vi "WriteVSChSingleIncoming.vi"(7 "IncomingFRActive?":bool, 8 "error in (no error)":errorcluster, 10 "Output Refs":T1[](array[typedef]) format="%.0x", 11 "Refnum in":refnum<k21>) -> (0 "error out":errorcluster, 1 "data":dbl[](array[numeric]), 3 "Refnum out":refnum<k21>)   [LabVIEW 2020, in "FlexRay Custom Device Engine.lvlib"]
uses:
  FlexRay Custom Device Engine.lvlib
  <vilib>/NI VeriStand/Custom Device API/Data Reference.ctl
  <vilib>/xnet/xnet.llb/XNET Read (Signal Single-point).vi
  <vilib>/NI VeriStand/Custom Device API/Global Data Refs.vi
  <vilib>/NI VeriStand/Custom Device API/Custom Device API.lvlib
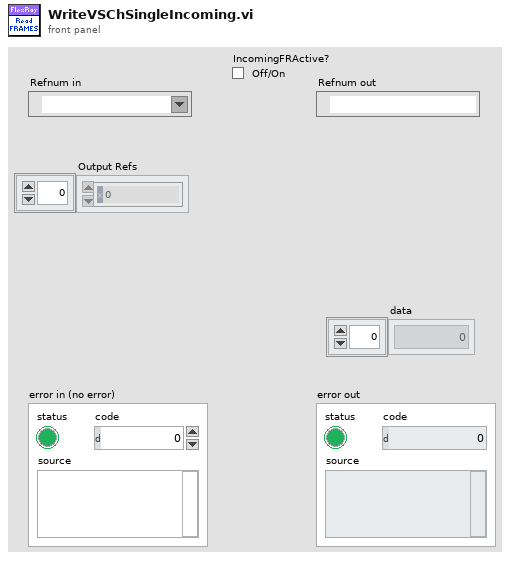
[diagram p1: front panel]
types:
  T1 = typedef "Custom Device API.lvlib/Data Reference.ctl" = i32
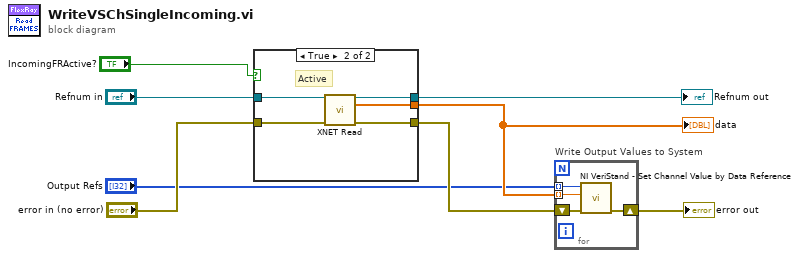
[diagram p0: block diagram]
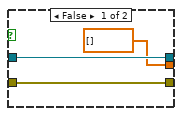
[diagram p2: hidden frame]
diagram:
  n1 = case shown="True" "IncomingFRActive?" {
    tunnel: [w10 w16] -> w2
    tunnel: [dbl[] [] ("data") w15] -> w3
    tunnel: "Refnum in" -> [w11 w14]
    tunnel: [w11 w13] -> w6
    tunnel: "error in (no error)" -> [w10 w12]
    frame False {
    }
    frame True {
      # "Active"
      n2 = call-poly <vilib>:"XNET Read.vi"("session in"=w14, "error in (no error)"=w12) -> ("session out"=w13:refnum<k21>, "data"=w15:dbl[], "error out"=w16:errorcluster)  [unwired: 11 in]
    }
  }
  "Refnum out" <- w6
  "data" <- w3
  n3 = for "Write Output Values to System" {
    shift-right: [w19] -> w4
    shift-left: w2 -> [w20]
    tunnel: "Output Refs" -> [w18] mode=indexing
    tunnel: w3 -> [w17] mode=indexing
    n4 = call <vilib>:"NI VeriStand - Set Channel Value by Data Reference.vi"("error in (no error)"=w20, "Value"=w17, "Data Reference in"=w18) -> ("error out"=w19:errorcluster)  [unwired: 8 in]
  }
  "error out" <- w4
